vi "SetNextPiplelineEnqueuer.vi"(8 "error in (no error)":errorcluster, 10 "NextPiplelineEnqueuer":refnum<class "Message Enqueuer.lvclass">, 11 "GRMActor in":refnum<class "GenericController.lvclass">) -> (0 "error out":errorcluster, 3 "GRMActor out":refnum<class "GenericController.lvclass">)   [LabVIEW 2020, in "GenericController.lvlib" / "GenericController.lvclass"]
uses:
  GenericController.lvclass
  <vilib>/ActorFramework/Message Enqueuer/Message Enqueuer.lvclass
  GenericController.lvclass/GenericController.ctl
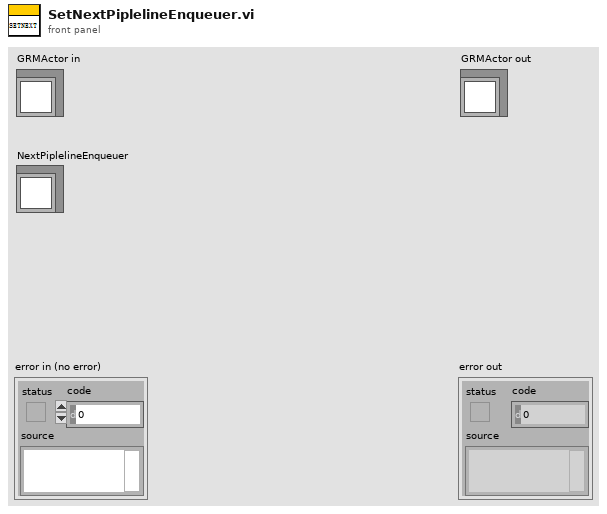
[diagram p1: front panel]
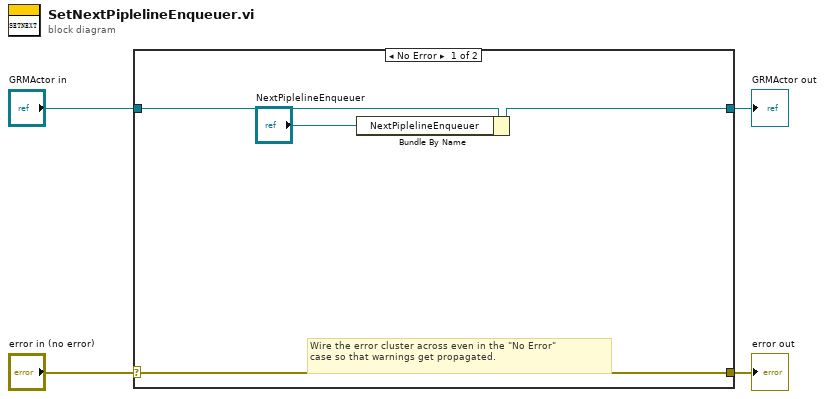
[diagram p0: block diagram]
diagram:
  n1 = case shown="No Error" "error in (no error)" {
    selector: "error in (no error)" -> [w7 w10]
    tunnel: [w7 w10] -> w3
    tunnel: [w6 w9] -> w1
    tunnel: "GRMActor in" -> [w8 w9]
    frame No Error {
      # "Wire the error cluster across even in the \"No Error\"\ncase so that warnings get propagated."
      n2 = Bundle By Name(cluster=w8, "NextPiplelineEnqueuer"="NextPiplelineEnqueuer") -> (w6:refnum<class "GenericController.lvclass">)
    }
    frame Error {
    }
  }
  "error out" <- w3
  "GRMActor out" <- w1
